vi "Write Numeric Bytes.vi"(8 "error in (no error)":errorcluster, 10 "Numeric Bytes":u8[](array[numeric]) format="%x", 11 "MessagePackNumeric in":refnum<class "MessagePackNumeric.lvclass">) -> (0 "error out":errorcluster, 3 "MessagePackNumeric out":refnum<class "MessagePackNumeric.lvclass">)   [LabVIEW 2020, in "MessagePack.lvlib" / "MessagePackNumeric.lvclass"]
uses:
  MessagePackNumeric.lvclass
  MessagePackNumeric.lvclass/MessagePackNumeric.ctl
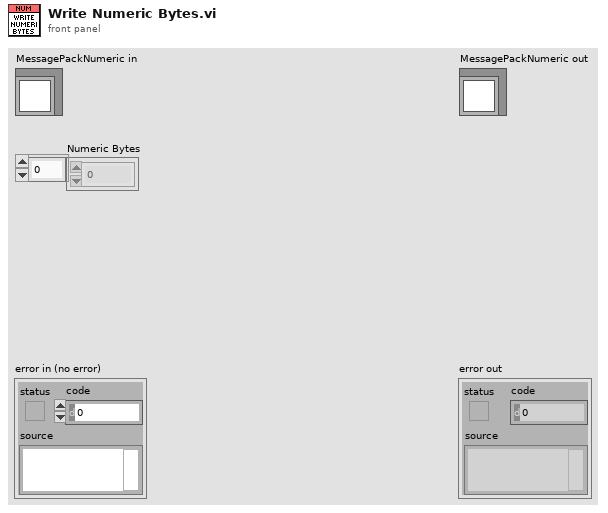
[diagram p1: front panel]
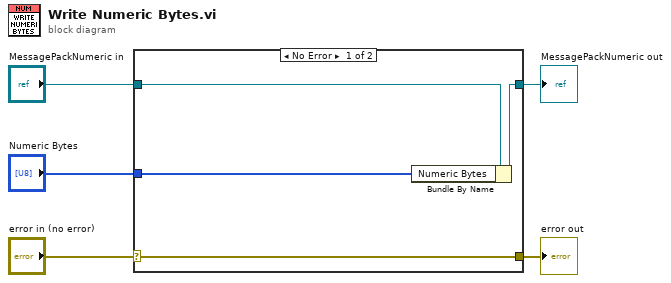
[diagram p0: block diagram]
diagram:
  n1 = case shown="No Error" "error in (no error)" {
    selector: "error in (no error)" -> [w9 w10]
    tunnel: [w9 w10] -> w4
    tunnel: [w7 w11] -> w2
    tunnel: "MessagePackNumeric in" -> [w8 w11]
    tunnel: "Numeric Bytes" -> [w6 _]
    frame No Error {
      n2 = Bundle By Name(cluster=w8, "Numeric Bytes"=w6) -> (w7:refnum<class "MessagePackNumeric.lvclass">)
    }
    frame Error {
    }
  }
  "error out" <- w4
  "MessagePackNumeric out" <- w2
